vi "LoopThroughGlobalVariables.vi"() -> ()   [LabVIEW 2019]
panel:
  out "Current Global File Path":path
  out "Global Variable Name":string
  out "Global Variable Value":string
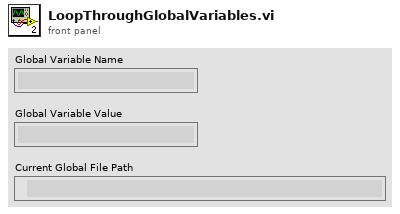
[diagram p1: front panel]
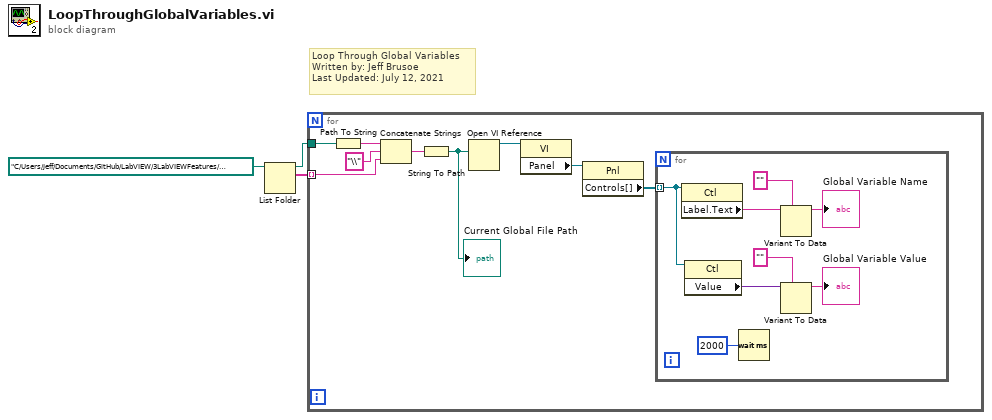
[diagram p0: block diagram]
diagram:
  # "Loop Through Global Variables\nWritten by: Jeff Brusoe\nLast Updated: July 12, 2021"
  n1 = List Folder(path=path "C:/Users/Jeff/Documents/GitHub/LabVIEW/3LabVIEWFeatures/LoopThroughGlobalVariables/Globals" ("vi path")) -> (path out=w1:path, filenames=w2:string[])  [unwired: 3 in, 2 out]
  n2 = for {
    tunnel: w2 -> [w7] mode=indexing
    tunnel: w1 -> [w9]
    n3 = Path To String(path=w9) -> (string=w8:string)
    n4 = Concatenate Strings(w8, "\\" ("string"), w7) -> (w5:string)
    n5 = String To Path(string=w5) -> (path=w4:path)
    "Current Global File Path" <- w4
    n6 = Open VI Reference(vi path=w4) -> (vi reference=w11:refnum<vi>)  [unwired: 5 in, 1 out]
    n7 = property class="VI"(reference=w11) -> ("Panel"=w10:refnum<vi>)  [unwired: 1 in, 2 out]
    n8 = property class="Pnl"(reference=w10) -> ("Controls[]"=w12:refnum<vi>[])  [unwired: 1 in, 2 out]
    n9 = for {
      tunnel: w12 -> [w14] mode=indexing
      n10 = property class="Ctl"(reference=w14) -> ("Label.Text"=w16:string)  [unwired: 1 in, 2 out]
      n11 = property class="Ctl"(reference=w14) -> ("Value"=w19:variant)  [unwired: 1 in, 2 out]
      n12 = Wait (ms)(milliseconds to wait=u32 2000) -> ()  [unwired: 1 out]
      n13 = Variant To Data(type="", Variant=w16) -> (data=→"Global Variable Name":string)  [unwired: 1 in, 1 out]
      n14 = Variant To Data(type="", Variant=w19) -> (data=→"Global Variable Value":string)  [unwired: 1 in, 1 out]
    }
  }
